vi "Force_1_R2.vi"() -> ()   [LabVIEW 2020]
uses:
  Support/Controls/Cmd_Mouse Popup.ctl
  Support/Controls/Clst_Initialize Input.ctl
  Support/Controls/Clst_Result inspec.ctl
  Support/Controls/Cmd_Var Data IO.ctl
  Variables/Global_Cal Info.vi
panel:
  out "Creep Test_ADJ":string[][](table) caption="2. 영점출력"
  in  "zero_30_ADJ":string[][](table) caption="2. 영점출력"
  in  "zero_300_ADJ":string[][](table) caption="2. 영점출력"
  in  "Measured_ADJ":string[][](table) caption="● 힘 측정기 지시값 (조정후)"
  out "지시단위":string="무차원"
  out "최대지시값":string
  in  "측정방향":string(combo)="인장"
  out "Creep Test":string[][](table) caption="2. 영점출력"
  in  "Case":enum16{"", "Case B", "Case D"}(ring)
  in  "zero_30":string[][](table) caption="2. 영점출력"
  in  "zero_300":string[][](table) caption="2. 영점출력"
  in  "Indicator info":string[][](table) caption="1. 사용 인디케이터"
  out "분해능":string
  out "표시방식":string
  in  "Spec 변경":bool
  in  "Random":bool
  out "Spec":string[][](table)
  out "제목":string
  out "에러 출력":errorcluster
  out "Condition":string[][](table) caption="3. 교정결과"
  in  "최소눈금":string(combo)
  out "단위":string
  out "최대용량":string
  in  "Measured":string[][](table) caption="● 힘 측정기 지시값"
  out "Load?":bool
  # "2. 영점출력 (조정후)"
  # "2. 영점출력"
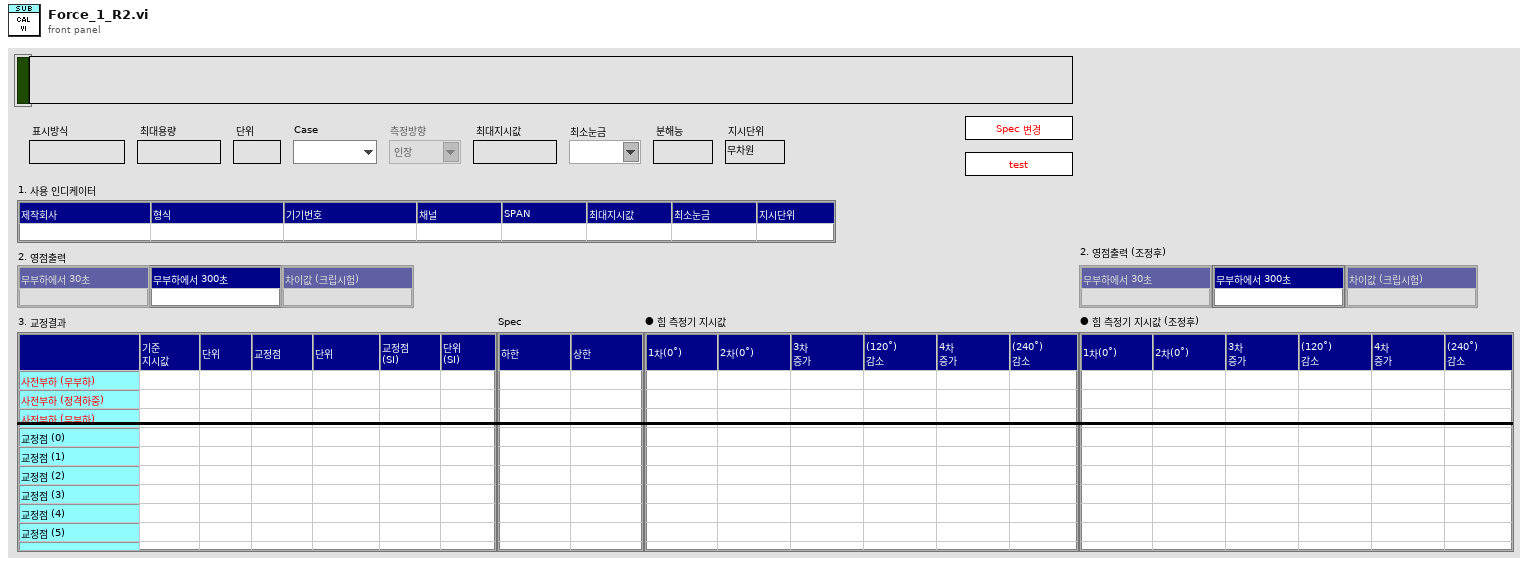
[diagram p1: front panel]
types:
  T1 = typedef "Cmd_Mouse Popup.ctl" = enum16{"활성화", "메뉴선택"}
  T2 = cluster{"Shift":bool, "Ctrl":bool, "Alt":bool, "Cmd":bool, "Opt":bool}
  T3 = enum8{"Enabled", "Disabled", "Disabled and Grayed Out"}
  T4 = typedef "Clst_Initialize Input.ctl" = cluster{"Initialize 1":cluster{"Condition":refnum<vi>[], "Spec":refnum<vi>[], "Measured":refnum<vi>[], "Resolution":refnum<vi>[], "Func_ext":string, "제목":refnum<vi>, "Measured_ADJ":refnum<vi>[]}, "Initialize 2":cluster{"문자열":refnum<vi>[], "콤보박스":refnum<vi>[], "링":refnum<vi>[], "열거형":refnum<vi>[], "테이블":refnum<vi>[], "여러열":refnum<vi>[], "디지털(DBL)":refnum<vi>[], "3D string":refnum<vi>[], "ctrl":refnum<vi>[], "boolean":refnum<vi>[]}}
  T5 = typedef "Clst_Result inspec.ctl" = cluster{"분해능":string, "문자열 1":string, "문자열 2":string, "숫자형 1":i32, "숫자형 2":i32, "숫자형 3":dbl, "문자배열 1D":string[], "문자배열 2D":string[][], "문자배열 3D":string[][][], "문자배열 4D":string[][][][], "불리언 1D":bool[]}
  T6 = typedef "Cmd_Var Data IO.ctl" = enum16{"Condition", "Condition Default", "Condition_Temp", "Resolution", "Resolution Default", "Resolution Old", "Spec", "Spec Default", "Spec Old", "Spec Temp", "Result", "Result2", "Result3", "Result_Temp", "Result_ADJ", "Result_ADJ2", "STD1", "STD2", "STD3", "STD4", "STD5", "STD Temp", "CMC", "CMC Default"}
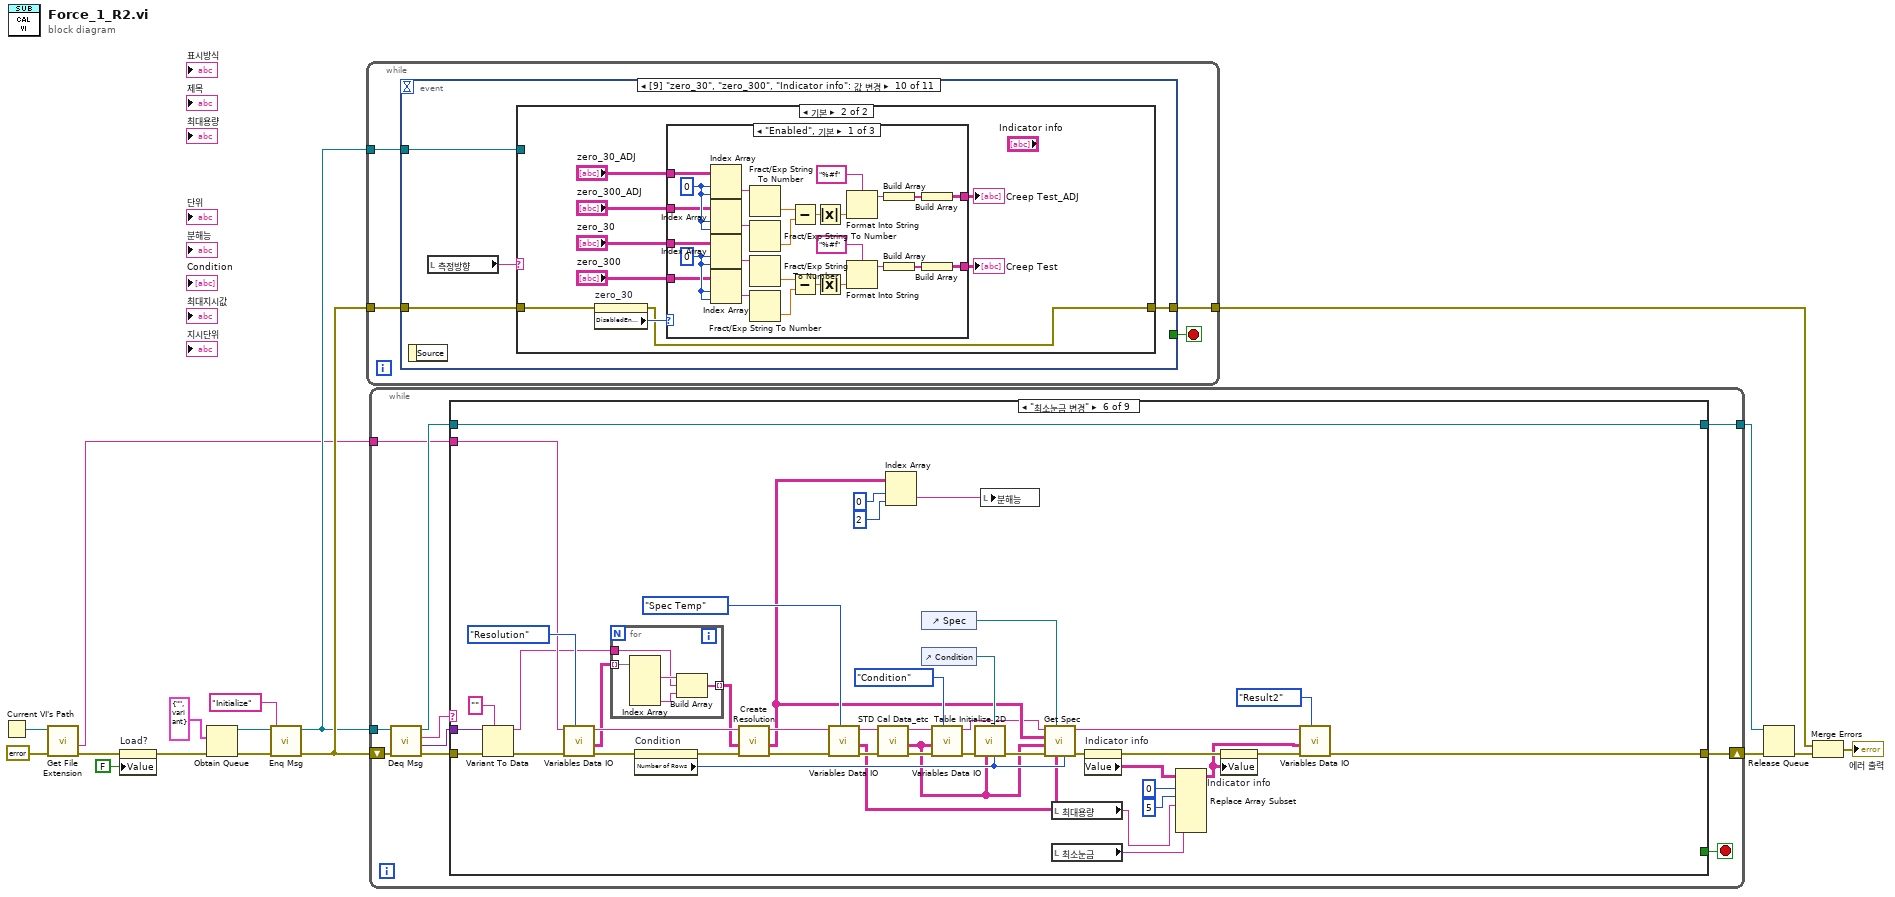
[diagram p0: block diagram]
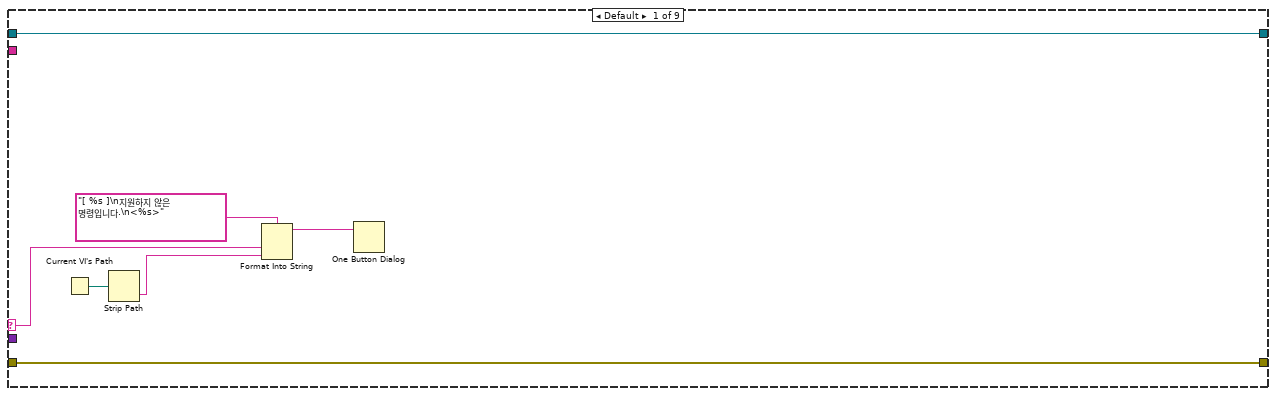
[diagram p2: hidden frame]
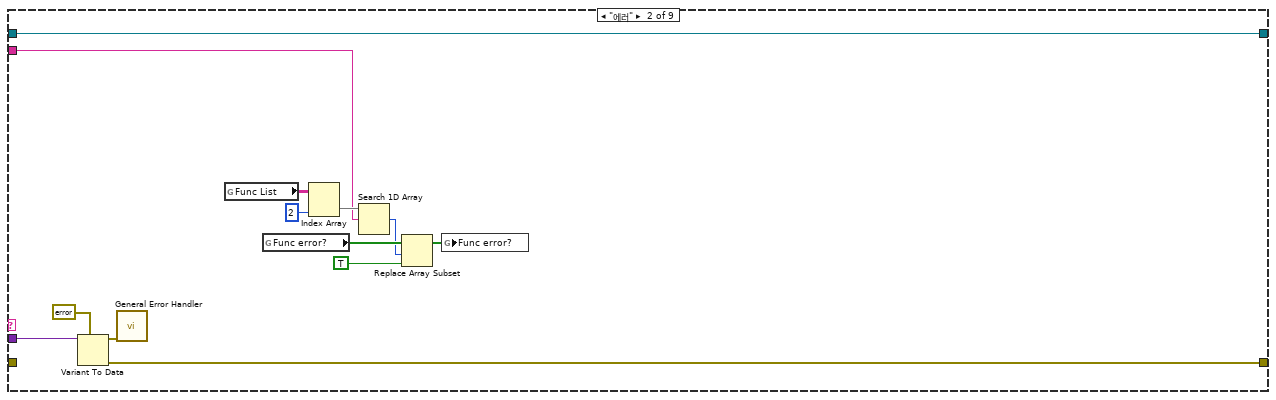
[diagram p3: hidden frame]
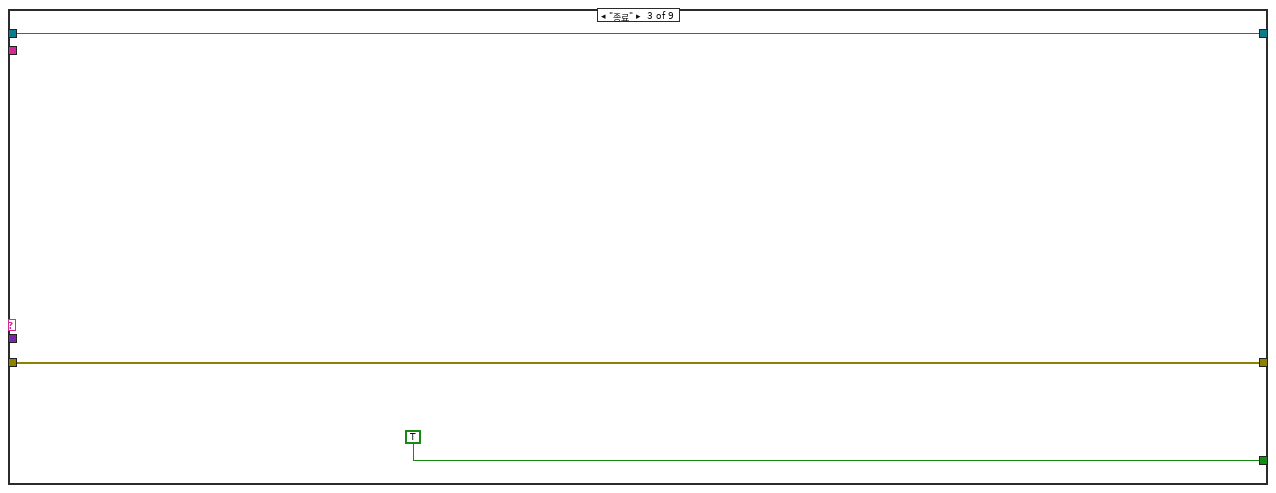
[diagram p4: hidden frame]
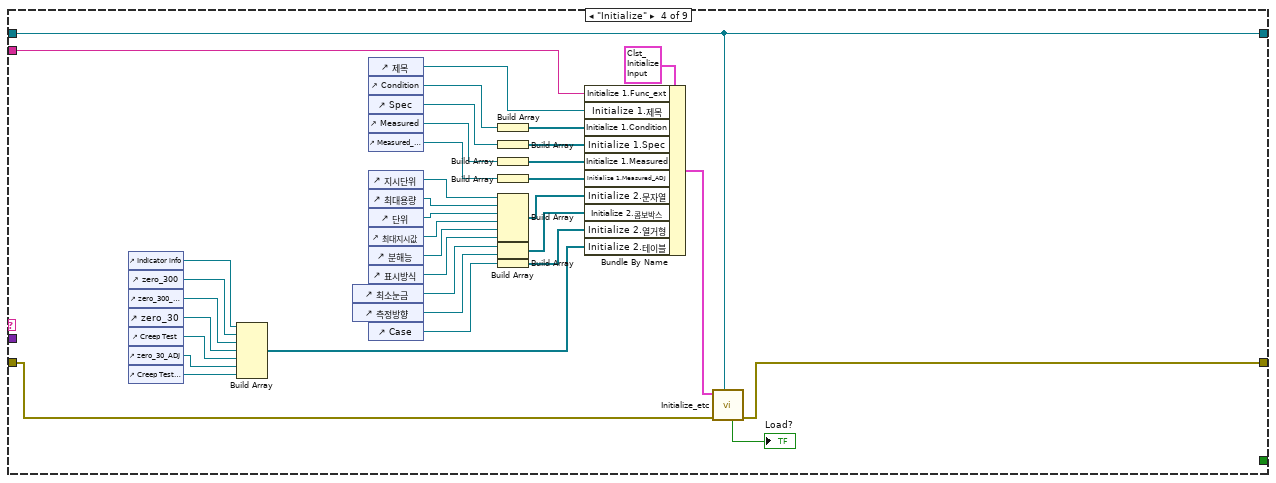
[diagram p5: hidden frame]
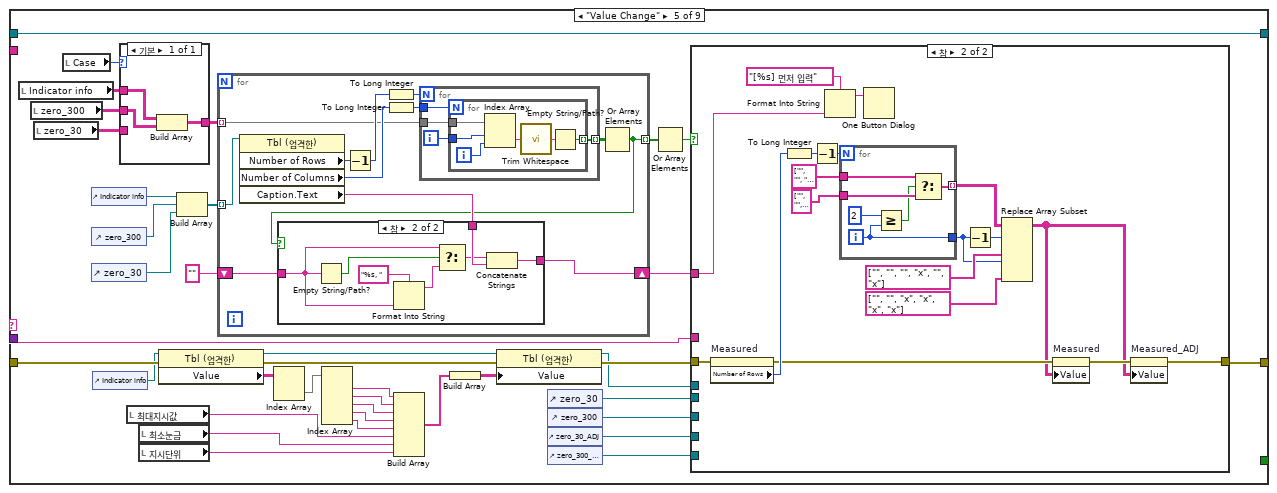
[diagram p6: hidden frame]
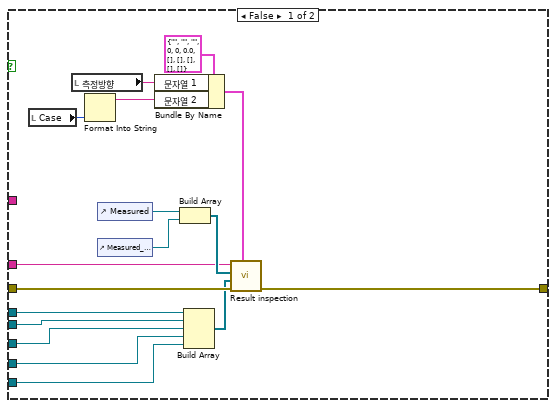
[diagram p7: hidden frame]
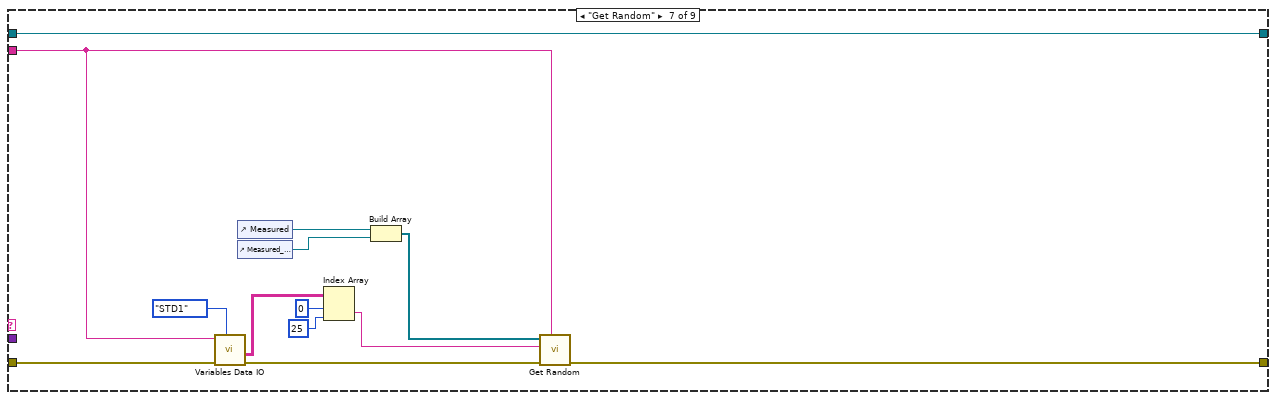
[diagram p9: hidden frame]
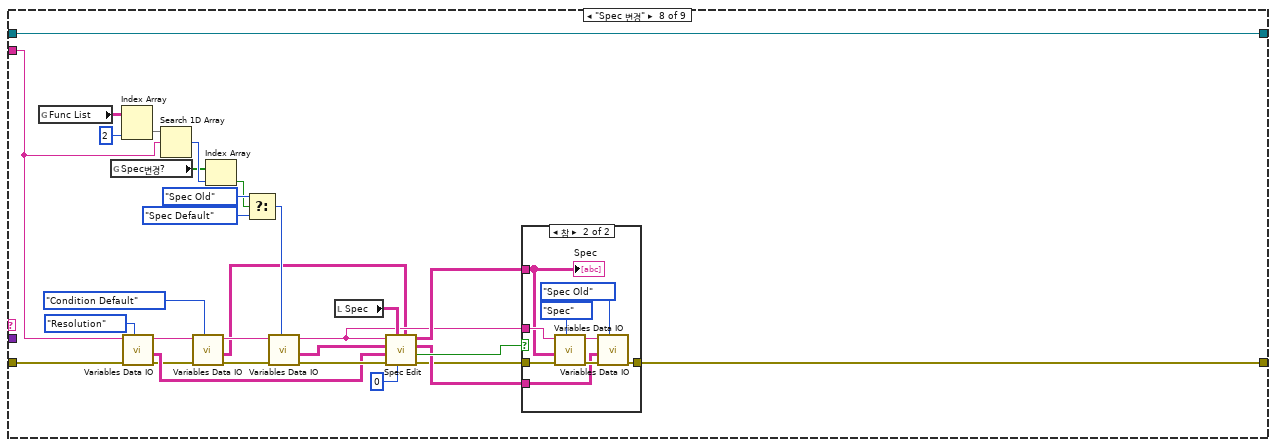
[diagram p10: hidden frame]
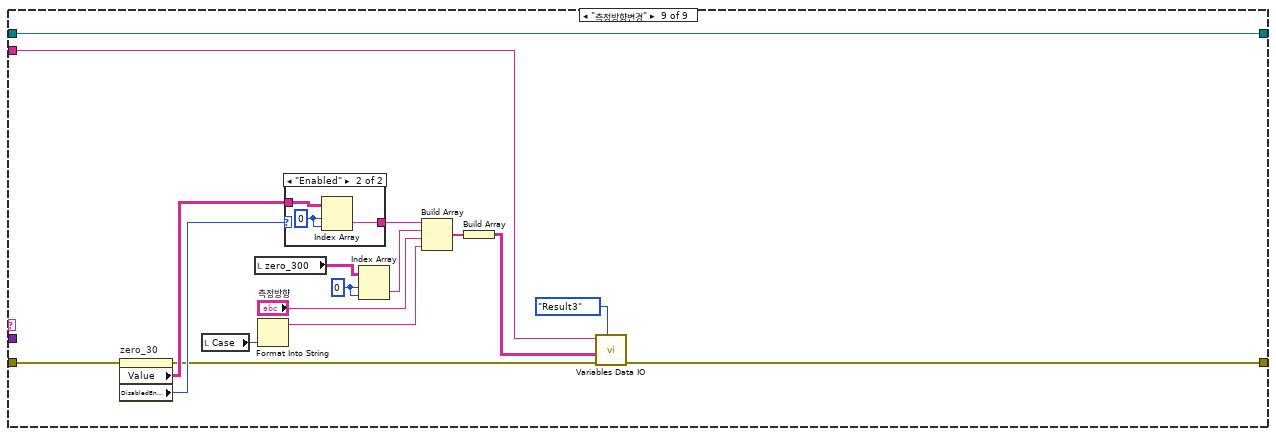
[diagram p12: hidden frame]
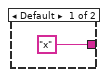
[diagram p13: hidden frame]
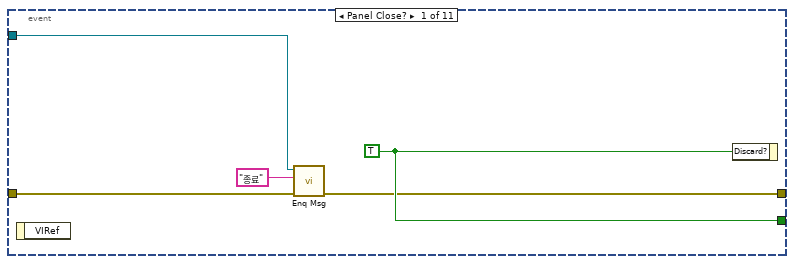
[diagram p14: hidden frame]
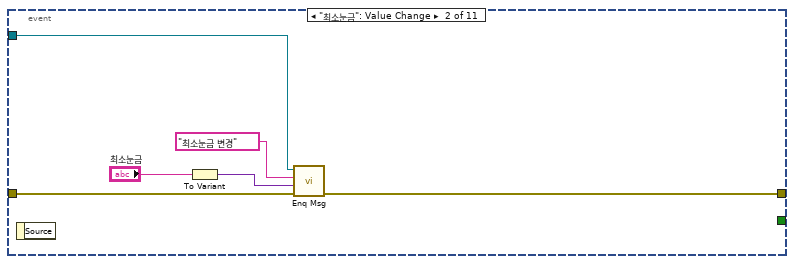
[diagram p15: hidden frame]
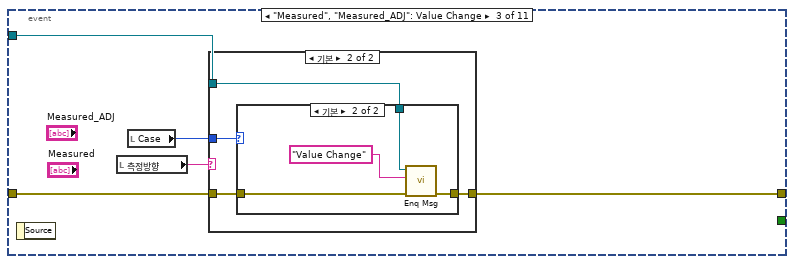
[diagram p16: hidden frame]
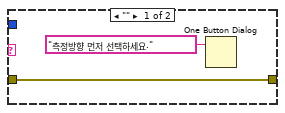
[diagram p17: hidden frame]
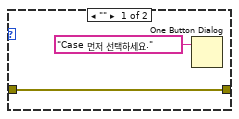
[diagram p18: hidden frame]
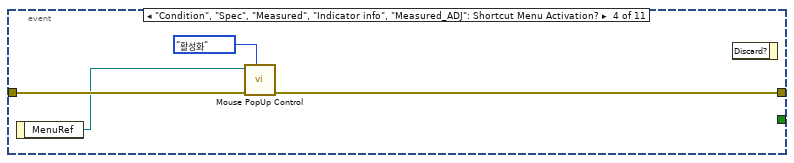
[diagram p19: hidden frame]
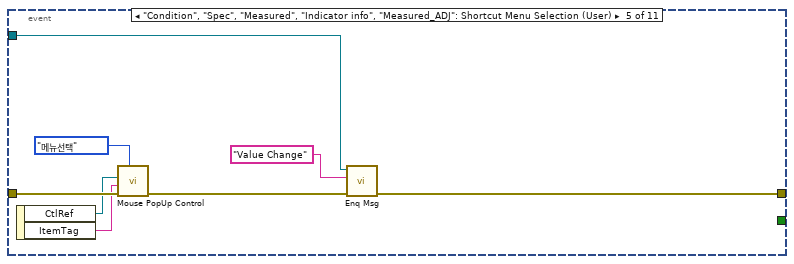
[diagram p20: hidden frame]
diagram:
  n1 = Current VI's Path() -> (path=w5:path)
  n2 = call <vilib>:"Get File Extension.vi"("error in (no error)"=errorcluster {"status"=FALSE, "code"=0, "source"=""} ("에러 상수"), "file"=w5) -> ("error out"=w3:errorcluster, "filename without extension"=w4:string)  [unwired: 5 in, 3 out]
  n3 = property on="Load?" class="Bool (엄격한)"(error in=w3, "Value"=FALSE ("Load?")) -> (error out=w2:errorcluster)  [unwired: 1 in, 1 out]
  n4 = Obtain Queue(element data type=cluster{"메세지":string, "값":variant} {"메세지"="", "값"=variant} ("Message Cluster"), error in (no error)=w2) -> (queue out=w14:refnum<queue>, error out=w16:errorcluster)  [unwired: 3 in, 1 out]
  n5 = call "Enq Msg.vi"("에러 입력(에러 없음)"=w16, "메세지"="Initialize", "큐 입력"=w14) -> ("에러 출력"=w15:errorcluster, "큐 출력"=w12:refnum<queue>)  [unwired: 7 in]
  n6 = while {
    tunnel: w15 -> [w19]
    tunnel: w12 -> [w20]
    tunnel: [w18] -> w9
    stop <- w21 stop-if-true
    n7 = event shown="[9] \"zero_30\", \"zero_300\", \"Indicator info\": 값 변경" {
      selector: _ -> [_ _ _ _ _ _ _ _ _ _ _]
      dyn-events: _ -> [_ _ _ _ _ _ _ _ _ _ _]
      timeout: _ -> [_ _ _ _ _ _ _ _ _ _ _]
      tunnel: [w26 _ _ _ _ _ _ _ _ _ _] -> w21
      tunnel: w20 -> [w24 w31 w36 _ w55 _ w69 w75 w81 w84 w124]
      tunnel: w19 -> [w25 w32 w37 w52 w60 w67 w70 w77 w80 w86 w126]
      tunnel: [w22 w29 w35 w51 w54 w66 w68 w76 w79 w85 w125] -> w18
      event Panel Close? {
        w26 = TRUE ("버림?")
        n8 = event-data() -> ()  [unwired: 1 in, 1 out]
        n9 = call "Enq Msg.vi"("에러 입력(에러 없음)"=w25, "메세지"="종료", "큐 입력"=w24) -> ("에러 출력"=w22:errorcluster)  [unwired: 7 in, 1 out]
        n10 = event-data("Discard?"=w26) -> ()  [unwired: 1 in, 1 out]
      }
      event "최소눈금": Value Change {
        n11 = event-data() -> ()  [unwired: 1 in, 1 out]
        n12 = To Variant(anything="최소눈금") -> (Variant=w27:variant)
        n13 = call "Enq Msg.vi"("에러 입력(에러 없음)"=w32, "값"=w27, "메세지"="최소눈금 변경", "큐 입력"=w31) -> ("에러 출력"=w29:errorcluster)  [unwired: 6 in, 1 out]
      }
      event "Measured", "Measured_ADJ": Value Change {
        n14 = event-data() -> ()  [unwired: 1 in, 1 out]
        n15 = local read "측정방향"() -> (w34:string)
        n16 = local read "Case"() -> (w33:enum16{"", "Case B", "Case D"})
        n17 = case shown="기본" w34 {
          tunnel: w37 -> [w39 w43]
          tunnel: w36 -> [_ w42]
          tunnel: [w39 w41] -> w35
          tunnel: w33 -> [_ w40]
          frame "" {
            n18 = One Button Dialog(message="측정방향 먼저 선택하세요." ("메시지")) -> ()  [unwired: 1 in, 1 out]
          }
          frame Default {
            n19 = case shown="기본" w40 {
              tunnel: w43 -> [w44 w49]
              tunnel: w42 -> [_ w48]
              tunnel: [w44 w46] -> w41
              frame "" {
                n20 = One Button Dialog(message="Case 먼저 선택하세요." ("메시지")) -> ()  [unwired: 1 in, 1 out]
              }
              frame Default {
                n21 = call "Enq Msg.vi"("에러 입력(에러 없음)"=w49, "메세지"="Value Change", "큐 입력"=w48) -> ("에러 출력"=w46:errorcluster)  [unwired: 7 in, 1 out]
              }
            }
          }
        }
      }
      event "Condition", "Spec", "Measured", "Indicator info", "Measured_ADJ": Shortcut Menu Activation? {
        n22 = event-data() -> ("MenuRef"=w50:refnum<k9>)  [unwired: 1 in]
        n23 = call "Mouse PopUp Control.vi"("type"=Cmd_Mouse_Popup."활성화", "error in"=w52, "메뉴 참조"=w50) -> ("error out"=w51:errorcluster)  [unwired: 8 in]
        n24 = event-data() -> ()  [unwired: 2 in, 1 out]
      }
      event "Condition", "Spec", "Measured", "Indicator info", "Measured_ADJ": Shortcut Menu Selection (User) {
        n25 = event-data() -> ("CtlRef"=w58:refnum<vi>, "ItemTag"=w59:string)  [unwired: 1 in]
        n26 = call "Mouse PopUp Control.vi"("type"=Cmd_Mouse_Popup."메뉴선택", "error in"=w60, "아이템 태그"=w59, "Tbl 참조 번호"=w58) -> ("error out"=w56:errorcluster)  [unwired: 7 in]
        n27 = call "Enq Msg.vi"("에러 입력(에러 없음)"=w56, "메세지"="Value Change", "큐 입력"=w55) -> ("에러 출력"=w54:errorcluster)  [unwired: 7 in, 1 out]
      }
      event "Measured", "Indicator info", "Condition", "Measured_ADJ": Key Down; "Measured", "Indicator info", "Condition", "Measured_ADJ": Key Repeat {
        n28 = event-data() -> ("PlatMods"=w62:T2, "ScanCode"=w65:i16, "Mods.Num Pad"=w64:bool, "CtlRef"=w63:refnum<vi>)  [unwired: 1 in]
        n29 = call "Cursor Control.vi"("플랫폼 조합키"=w62, "참조"=w63, "Num Pad"=w64, "ScanCode"=w65, "error in"=w67) -> ("error out"=w66:errorcluster)  [unwired: 5 in, 1 out]
      }
      event "Random": Value Change {
        n30 = event-data() -> ()  [unwired: 1 in, 1 out]
        n31 = call "Enq Msg.vi"("에러 입력(에러 없음)"=w70, "메세지"="Get Random", "큐 입력"=w69) -> ("에러 출력"=w72:errorcluster, "큐 출력"=w73:refnum<queue>)  [unwired: 7 in]
        n32 = call "Enq Msg.vi"("에러 입력(에러 없음)"=w72, "메세지"="Value Change", "큐 입력"=w73) -> ("에러 출력"=w68:errorcluster)  [unwired: 7 in, 1 out]
      }
      event "Spec 변경": Value Change {
        n33 = event-data() -> ()  [unwired: 1 in, 1 out]
        n34 = call "Enq Msg.vi"("에러 입력(에러 없음)"=w77, "메세지"="Spec 변경", "큐 입력"=w75) -> ("에러 출력"=w76:errorcluster)  [unwired: 7 in, 1 out]
      }
      event "Case": Value Change {
        n35 = event-data() -> ()  [unwired: 1 in, 1 out]
        n36 = call "Enq Msg.vi"("에러 입력(에러 없음)"=w80, "메세지"="Value Change", "큐 입력"=w81) -> ("에러 출력"=w79:errorcluster)  [unwired: 7 in, 1 out]
      }
      event "zero_30", "zero_300", "Indicator info": Value Change {
        n37 = event-data() -> ()  [unwired: 1 in, 1 out]
        n38 = local read "측정방향"() -> (w83:string)
        n39 = case shown="기본" w83 {
          tunnel: w86 -> [w88 w95]
          tunnel: [w88 w92] -> w85
          tunnel: w84 -> [_ _]
          frame "" {
            n40 = One Button Dialog(message="측정방향 먼저 선택하세요." ("메시지")) -> ()  [unwired: 1 in, 1 out]
          }
          frame Default {
            n41 = property on="zero_30" class="Tbl (엄격한)"(error in=w95) -> (error out=w92:errorcluster, "DisabledEnum"=w94:T3)  [unwired: 1 in, 1 out]
            n42 = case shown="\"Enabled\", 기본" w94 {
              tunnel: "zero_30" -> [w122 _ _]
              tunnel: "zero_300" -> [w120 _ _]
              tunnel: [w112 _ _] -> w93
              tunnel: "zero_30_ADJ" -> [w100 _ _]
              tunnel: "zero_300_ADJ" -> [w99 _ _]
              tunnel: [w98 _ _] -> w89
              frame "Enabled", Default {
                w101 = 0 ("인덱스 (행)")
                w123 = 0 ("인덱스 (행)")
                n43 = Index Array(array=w100, index (row)=w101, index (col)=w101) -> (element=w105:string)
                n44 = Index Array(array=w99, index (row)=w101, index (col)=w101) -> (element=w106:string)
                n45 = Index Array(array=w122, index (row)=w123, index (col)=w123) -> (element=w117:string)
                n46 = Index Array(array=w120, index (row)=w123, index (col)=w123) -> (element=w116:string)
                n47 = Fract/Exp String To Number(string=w105) -> (number=w102:dbl)  [unwired: 3 in, 1 out]
                n48 = Fract/Exp String To Number(string=w106) -> (number=w103:dbl)  [unwired: 3 in, 1 out]
                n49 = Fract/Exp String To Number(string=w117) -> (number=w121:dbl)  [unwired: 3 in, 1 out]
                n50 = Fract/Exp String To Number(string=w116) -> (number=w119:dbl)  [unwired: 3 in, 1 out]
                n51 = Subtract(x=w102, y=w103) -> (x-y=w104:dbl)
                n52 = Subtract(x=w121, y=w119) -> (x-y=w118:dbl)
                n53 = Absolute Value(x=w104) -> (abs(x)=w110:dbl)
                n54 = Absolute Value(x=w118) -> (abs(x)=w111:dbl)
                n55 = Format Into String(format string="%#f" ("포맷 문자열"), w110) -> (resulting string=w108:string)  [unwired: 2 in, 1 out]
                n56 = Format Into String(format string="%#f" ("포맷 문자열"), w111) -> (resulting string=w114:string)  [unwired: 2 in, 1 out]
                n57 = Build Array(w108) -> (w109:string[])
                n58 = Build Array(w114) -> (w113:string[])
                n59 = Build Array(w109) -> (w98:string[][])
                n60 = Build Array(w113) -> (w112:string[][])
              }
              frame "Disabled" {
              }
              frame "Disabled and Grayed Out" {
              }
            }
            "Creep Test" <- w93
            "Creep Test_ADJ" <- w89
          }
        }
      }
      event "측정방향": Value Change {
        n61 = event-data() -> ()  [unwired: 1 in, 1 out]
        n62 = call "Enq Msg.vi"("에러 입력(에러 없음)"=w126, "메세지"="측정방향변경", "큐 입력"=w124) -> ("에러 출력"=w125:errorcluster)  [unwired: 7 in, 1 out]
      }
    }
  }
  n63 = while {
    shift-right: [w137] -> w11
    shift-left: w15 -> [w136]
    tunnel: w12 -> [w134]
    tunnel: [w129] -> w10
    tunnel: w4 -> [w128]
    stop <- w130 stop-if-true
    n64 = call "Deq Msg.vi"("에러 입력(에러 없음)"=w136, "큐 입력"=w134) -> ("에러 출력"=w135:errorcluster, "값"=w131:variant, "메세지"=w133:string, "큐 출력"=w132:refnum<queue>)  [unwired: 6 in]
    n65 = case shown="\"최소눈금 변경\"" w133 {
      selector: w133 -> [w140 _ _ _ _ _ _ _ _]
      tunnel: w135 -> [w144 _ w160 w175 w216 w352 w366 w381 w414]
      tunnel: [w144 w154 w160 w180 w225 w316 w369 w382 w426] -> w137
      tunnel: w132 -> [w143 w153 w158 w184 w234 w353 w371 w401 w428]
      tunnel: w131 -> [_ w155 _ _ _ w351 _ _ _]
      tunnel: [_ _ TRUE ("버림?") _ _ _ _ _ _] -> w130
      tunnel: [w143 w153 w158 w184 w234 w353 w371 w401 w428] -> w129
      tunnel: w128 -> [_ w145 _ w179 w224 w347 w367 w380 w425]
      frame Default {
        n66 = Current VI's Path() -> (path=w139:path)
        n67 = Strip Path(path=w139) -> (name=w138:string)  [unwired: 1 out]
        n68 = Format Into String(format string="[ %s ]\n지원하지 않은 명령입니다.\n<%s>" ("메시지"), w140, w138) -> (resulting string=w141:string)  [unwired: 2 in, 1 out]
        n69 = One Button Dialog(message=w141) -> ()  [unwired: 1 in, 1 out]
      }
      frame "에러" {
        n70 = Variant To Data(type=errorcluster {"status"=FALSE, "code"=0, "source"=""} ("에러 출력"), Variant=w155) -> (data=w157:errorcluster, error out=w154:errorcluster)  [unwired: 1 in]
        n71 = call <vilib>:"General Error Handler.vi"("error in (no error)"=w157) -> ()  [unwired: 10 in, 5 out]
        n72 = global read "Global_Cal Info.vi" "Func List"() -> (w151:string[][])
        n73 = global read "Global_Cal Info.vi" "Func error?"() -> (w148:bool[])
        n74 = Index Array(array=w151, index (col)=2 ("비활성화된 인덱스 (열)")) -> (element=w150:string[])  [unwired: 1 in]
        n75 = Search 1D Array(1D array=w150, element=w145) -> (index of element=w147:i32)  [unwired: 1 in]
        n76 = Replace Array Subset(array=w148, new element=TRUE ("새 원소/부분배열"), index=w147) -> (w146:bool[])
        n77 = global write "Global_Cal Info.vi" "Func error?"(w146) -> ()
      }
      frame "종료" {
      }
      frame "Initialize" {
        n78 = control-ref of="Indicator info"() -> (w174:refnum<vi>)
        n79 = control-ref of="zero_300"() -> (w173:refnum<vi>)
        n80 = control-ref of="zero_300_ADJ"() -> (w165:refnum<vi>)
        n81 = control-ref of="zero_30"() -> (w164:refnum<vi>)
        n82 = control-ref of="Creep Test"() -> (w163:refnum<vi>)
        n83 = control-ref of="zero_30_ADJ"() -> (w162:refnum<vi>)
        n84 = control-ref of="Creep Test_ADJ"() -> (w166:refnum<vi>)
        n85 = Build Array(w174, w173, w165, w164, w163, w162, w166) -> (w172:refnum<vi>[])
        n86 = control-ref of="최소눈금"() -> (w190:refnum<vi>)
        n87 = control-ref of="측정방향"() -> (w171:refnum<vi>)
        n88 = control-ref of="제목"() -> (w188:refnum<vi>)
        n89 = control-ref of="Condition"() -> (w183:refnum<vi>)
        n90 = control-ref of="Spec"() -> (w182:refnum<vi>)
        n91 = control-ref of="Measured"() -> (w192:refnum<vi>)
        n92 = control-ref of="Measured_ADJ"() -> (w167:refnum<vi>)
        n93 = control-ref of="지시단위"() -> (w169:refnum<vi>)
        n94 = control-ref of="최대용량"() -> (w187:refnum<vi>)
        n95 = control-ref of="단위"() -> (w178:refnum<vi>)
        n96 = control-ref of="최대지시값"() -> (w186:refnum<vi>)
        n97 = control-ref of="분해능"() -> (w181:refnum<vi>)
        n98 = control-ref of="표시방식"() -> (w170:refnum<vi>)
        n99 = control-ref of="Case"() -> (w177:refnum<vi>)
        n100 = Build Array(w183) -> (w194:refnum<vi>[])
        n101 = Build Array(w182) -> (w185:refnum<vi>[])
        n102 = Build Array(w192) -> (w193:refnum<vi>[])
        n103 = Build Array(w167) -> (w168:refnum<vi>[])
        n104 = Build Array(w169, w187, w178, w186, w181, w170) -> (w191:refnum<vi>[])
        n105 = Build Array(w190, w171) -> (w189:refnum<vi>[])
        n106 = Build Array(w177) -> (w176:refnum<vi>[])
        n107 = Bundle By Name(cluster=T4 {"Initialize 1"={"Condition"=[], "Spec"=[], "Measured"=[], "Resolution"=[], "Func_ext"="", "제목"=refnum, "Measured_ADJ"=[]}, "Initialize 2"={"문자열"=[], "콤보박스"=[], "링"=[], "열거형"=[], "테이블"=[], "여러열"=[], "디지털(DBL)"=[], "3D string"=[], "ctrl"=[], "boolean"=[]}} ("입력 클러스터"), "Initialize 1.Func_ext"=w179, "Initialize 1.제목"=w188, "Initialize 1.Condition"=w194, "Initialize 1.Spec"=w185, "Initialize 1.Measured"=w193, "Initialize 1.Measured_ADJ"=w168, "Initialize 2.문자열"=w191, "Initialize 2.콤보박스"=w189, "Initialize 2.열거형"=w176, "Initialize 2.테이블"=w172) -> (w195:T4)
        n108 = call "Initialize_etc.vi"("큐 입력"=w184, "error in"=w175, "입력 클러스터"=w195) -> ("error out"=w180:errorcluster, "Load?"=→"Load?":bool)  [unwired: 6 in, 1 out]
      }
      frame "Value Change" {
        n109 = local read "Indicator info"() -> (w217:string[][])
        n110 = local read "zero_300"() -> (w220:string[][])
        n111 = local read "zero_30"() -> (w221:string[][])
        n112 = local read "Case"() -> (w232:enum16{"", "Case B", "Case D"})
        n113 = control-ref of="Indicator info"() -> (w230:refnum<vi>)
        n114 = control-ref of="zero_300"() -> (w229:refnum<vi>)
        n115 = control-ref of="zero_30"() -> (w228:refnum<vi>)
        n116 = control-ref of="Indicator info"() -> (w212:refnum<vi>)
        n117 = case shown="기본" w232 {
          tunnel: w217 -> [w278]
          tunnel: w220 -> [w277]
          tunnel: w221 -> [_]
          tunnel: [w276] -> w231
          frame 기본 {
            n118 = Build Array(w278, w277) -> (w276:string[][][])
          }
        }
        n119 = local read "최대지시값"() -> (w203:string)
        n120 = local read "최소눈금"() -> (w202:string)
        n121 = local read "지시단위"() -> (w201:string)
        n122 = property on="프로퍼티 노드" class="Tbl (엄격한)"(reference=w212, error in=w216) -> (reference out=w213:refnum<vi>, error out=w215:errorcluster, "Value"=w210:string[][])
        n123 = Build Array(w230, w229, w228) -> (w227:refnum<vi>[])
        n124 = for {
          tunnel: w227 -> [w290] mode=indexing
          tunnel: w231 -> [w286] mode=indexing
          tunnel: [w279] -> w233 mode=indexing
          shift-right: [w283] -> w222
          shift-left: "" -> [w284]
          n125 = property on="프로퍼티 노드" class="Tbl (엄격한)"(reference=w290) -> ("Number of Rows"=w289:u32, "Number of Columns"=w288:u32, "Caption.Text"=w285:string)  [unwired: 1 in, 2 out]
          n126 = Decrement(x=w289) -> (x-1=w287:u32)
          n127 = To Long Integer(number=w287) -> (32bit integer=w282:i32)
          n128 = To Long Integer(number=w288) -> (32bit integer=w281:i32)
          n129 = for {
            N: w282 -> [_]
            tunnel: w286 -> [w301]
            tunnel: w281 -> [w302]
            tunnel: [w300] -> w280 mode=indexing
            i -> [w299]
            n130 = for {
              N: w302 -> [_]
              tunnel: w301 -> [w306]
              tunnel: [w307] -> w300 mode=indexing
              tunnel: w299 -> [w304]
              i -> [w303]
              n131 = Index Array(array=w306, index (row)=w304, index (col)=w303) -> (element=w305:string)
              n132 = call <vilib>:"Trim Whitespace.vi"("string"=w305) -> ("trimmed string"=w308:string)  [unwired: 1 in]
              n133 = Empty String/Path?(string/path=w308) -> (empty?=w307:bool)
            }
          }
          n134 = Or Array Elements(Boolean array=w280) -> (logical OR=w279:bool)
          n135 = case shown="참" w279 {
            tunnel: w285 -> [_ w298]
            tunnel: w284 -> [w291 w297]
            tunnel: [w291 w296] -> w283
            frame False {
            }
            frame True {
              n136 = Empty String/Path?(string/path=w297) -> (empty?=w295:bool)
              n137 = Format Into String(format string="%s, " ("포맷 문자열"), w297) -> (resulting string=w293:string)  [unwired: 2 in, 1 out]
              n138 = Select(t=w297, s=w295, f=w293) -> (s? t:f=w292:string)
              n139 = Concatenate Strings(w292, w298) -> (w296:string)
            }
          }
        }
        n140 = Index Array(array=w210) -> (element=w209:string[])  [unwired: 2 in]
        n141 = Index Array(array=w209) -> (element #1=w208:string, element #2=w207:string, element #3=w206:string, element #4=w205:string, element #5=w204:string)  [unwired: 5 in]
        n142 = Build Array(w208, w207, w206, w205, w204, w203, w202, w201) -> (w200:string[])
        n143 = Build Array(w200) -> (w199:string[][])
        n144 = property on="프로퍼티 노드" class="Tbl (엄격한)"(reference=w213, error in=w215, "Value"=w199) -> (reference out=w211:refnum<vi>, error out=w214:errorcluster)
        n145 = control-ref of="zero_30"() -> (w219:refnum<vi>)
        n146 = control-ref of="zero_300"() -> (w218:refnum<vi>)
        n147 = control-ref of="zero_30_ADJ"() -> (w198:refnum<vi>)
        n148 = control-ref of="zero_300_ADJ"() -> (w197:refnum<vi>)
        n149 = Or Array Elements(Boolean array=w233) -> (logical OR=w223:bool)
        n150 = case shown="참" w223 {
          tunnel: [w251 w253] -> w225
          tunnel: w214 -> [w250 w266]
          tunnel: w224 -> [w247 _]
          tunnel: w222 -> [_ w267]
          tunnel: w211 -> [w246 _]
          tunnel: w219 -> [w245 _]
          tunnel: w218 -> [w244 _]
          tunnel: w198 -> [w236 _]
          tunnel: w197 -> [w235 _]
          frame False {
            n151 = local read "Case"() -> (w239:enum16{"", "Case B", "Case D"})
            n152 = local read "측정방향"() -> (w240:string)
            n153 = Format Into String(w239) -> (resulting string=w238:string)  [unwired: 3 in, 1 out]
            n154 = control-ref of="Measured"() -> (w249:refnum<vi>)
            n155 = control-ref of="Measured_ADJ"() -> (w237:refnum<vi>)
            n156 = Bundle By Name(cluster=T5 {"분해능"="", "문자열 1"="", "문자열 2"="", "숫자형 1"=0, "숫자형 2"=0, "숫자형 3"=0.0, "문자배열 1D"=[], "문자배열 2D"=[], "문자배열 3D"=[], "문자배열 4D"=[], "불리언 1D"=[]} ("입력 클러스터"), "문자열 1"=w240, "문자열 2"=w238) -> (w241:T5)
            n157 = Build Array(w249, w237) -> (w248:refnum<vi>[])
            n158 = Build Array(w246, w245, w244, w236, w235) -> (w243:refnum<vi>[])
            n159 = call "Result inspection.vi"("입력 클러스터"=w241, "error in"=w250, "Ref. Data (excluded)"=w243, "Ref. Data (Inspection)"=w248, "Func ext"=w247) -> ("error out"=w251:errorcluster)  [unwired: 3 in, 3 out]
          }
          frame True {
            n160 = property on="Measured" class="Tbl (엄격한)"(error in=w266) -> (error out=w255:errorcluster, "Number of Rows"=w256:u32)  [unwired: 1 in, 1 out]
            n161 = To Long Integer(number=w256) -> (32bit integer=w264:i32)
            n162 = Decrement(x=w264) -> (x-1=w265:i32)
            n163 = Format Into String(format string="[%s] 먼저 입력" ("포맷 문자열"), w267) -> (resulting string=w269:string)  [unwired: 2 in, 1 out]
            n164 = for {
              N: w265 -> [_]
              tunnel: [w272] -> w257 mode=indexing
              tunnel: [w275] -> w259
              tunnel: string[] ["", "", "", "", "", ""] -> [w274]
              tunnel: string[] ["", "", "", "ⅹ", "ⅹ", "ⅹ"] -> [w273]
              i -> [w275]
              n165 = Greater Or Equal?(x=2, y=w275) -> (x >= y?=w271:bool)
              n166 = Select(t=w273, s=w271, f=w274) -> (s? t:f=w272:string[])
            }
            n167 = One Button Dialog(message=w269) -> ()  [unwired: 1 in, 1 out]
            n168 = Decrement(x=w259) -> (x-1=w260:i32)
            n169 = Replace Array Subset(array=w257, new element #1=string[] ["", "", "", "ⅹ", "", "ⅹ"], index (row) #1=w260, new element #2=string[] ["", "", "ⅹ", "ⅹ", "ⅹ", "ⅹ"], index (row) #2=w259) -> (w252:string[][])  [unwired: 2 in]
            n170 = property on="Measured" class="Tbl (엄격한)"(error in=w255, "Value"=w252) -> (error out=w254:errorcluster)  [unwired: 1 in, 1 out]
            n171 = property on="Measured_ADJ" class="Tbl (엄격한)"(error in=w254, "Value"=w252) -> (error out=w253:errorcluster)  [unwired: 1 in, 1 out]
          }
        }
      }
      frame "최소눈금 변경" {
        n172 = Variant To Data(error in=w352, type="", Variant=w351) -> (data=w345:string, error out=w346:errorcluster)
        n173 = call "Variables Data IO.vi"("Select"=Cmd_Var_Data_IO."Resolution", "error in"=w346, "Func_ext"=w347) -> ("error out"=w331:errorcluster, "Data Out"=w344:string[][], "Func_ext Out"=w348:string)  [unwired: 6 in]
        n174 = for {
          tunnel: w344 -> [w358] mode=indexing
          tunnel: w345 -> [w356]
          tunnel: [w354] -> w343 mode=indexing
          n175 = Index Array(array=w358) -> (element #1=w357:string, element #4=w355:string)  [unwired: 4 in, 2 out]
          n176 = Build Array(w357, w356, w355) -> (w354:string[])
        }
        n177 = property on="Condition" class="Tbl (엄격한)"(error in=w331) -> (error out=w330:errorcluster, "Number of Rows"=w313:u32)  [unwired: 1 in, 1 out]
        n178 = call "Create Resolution.vi"("에러 입력(에러 없음)"=w330, "Resolution"=w343, "Func_ext"=w348) -> ("에러 출력"=w335:errorcluster, "Resolution Out"=w310:string[][], "Func_ext 출력"=w334:string)  [unwired: 6 in]
        n179 = call "Variables Data IO.vi"("Select"=Cmd_Var_Data_IO."Spec Temp", "error in"=w335, "Func_ext"=w334) -> ("error out"=w333:errorcluster, "Data Out"=w312:string[][], "Func_ext Out"=w332:string)  [unwired: 6 in]
        n180 = call "STD Cal Data_etc.vi"("error in"=w333, "Func_ext"=w332) -> ("error out"=w340:errorcluster, "Data Out"=w311:string[][], "Func_ext Out"=w341:string)  [unwired: 5 in, 2 out]
        n181 = Index Array(array=w310, index (row)=0 ("인덱스 (행)"), index (col)=2 ("비활성화된 인덱스 (열)")) -> (element=w327:string)
        n182 = control-ref of="Spec"() -> (w337:refnum<vi>)
        n183 = control-ref of="Condition"() -> (w326:refnum<vi>)
        n184 = call "Variables Data IO.vi"("Select"=Cmd_Var_Data_IO."Condition", "error in"=w340, "Data In"=w311, "Func_ext"=w341) -> ("error out"=w339:errorcluster, "Func_ext Out"=w309:string)  [unwired: 5 in, 1 out]
        n185 = call "Table Initialize_2D.vi"("행의 개수"=w313, "Table Ref"=w326, "Value"=w311, "에러 입력"=w339) -> ("에러 출력"=w342:errorcluster)  [unwired: 5 in, 2 out]
        n186 = local write "분해능"(w327) -> ()
        n187 = call "Get Spec.vi"("NumRows"=w313, "Spec in"=w312, "Spec Ref."=w337, "error in"=w342, "Condition in"=w311, "Resolution in"=w310, "Func_ext"=w309) -> ("error out"=w319:errorcluster, "Func_ext Out"=w315:string)  [unwired: 3 out]
        n188 = local read "최대용량"() -> (w322:string)
        n189 = local read "최소눈금"() -> (w320:string)
        n190 = property on="Indicator info" class="Tbl (엄격한)"(error in=w319) -> (error out=w325:errorcluster, "Value"=w324:string[][])  [unwired: 1 in, 1 out]
        n191 = Replace Array Subset(array=w324, new element #1=w322, index (row) #1=0 ("비활성화된 인덱스 (행)"), index (col) #1=5 ("비활성화된 인덱스 (열)"), new element #2=w320) -> (w314:string[][])  [unwired: 2 in]
        n192 = property on="Indicator info" class="Tbl (엄격한)"(error in=w325, "Value"=w314) -> (error out=w317:errorcluster)  [unwired: 1 in, 1 out]
        n193 = call "Variables Data IO.vi"("Select"=Cmd_Var_Data_IO."Result2", "error in"=w317, "Data In"=w314, "Func_ext"=w315) -> ("error out"=w316:errorcluster)  [unwired: 5 in, 2 out]
      }
      frame "Get Random" {
        n194 = call "Variables Data IO.vi"("Select"=Cmd_Var_Data_IO."STD1", "error in"=w366, "Func_ext"=w367) -> ("error out"=w365:errorcluster, "Data Out"=w363:string[][])  [unwired: 6 in, 1 out]
        n195 = control-ref of="Measured"() -> (w368:refnum<vi>)
        n196 = control-ref of="Measured_ADJ"() -> (w359:refnum<vi>)
        n197 = Index Array(array=w363, index (row)=0 ("인덱스 (행)"), index (col)=25 ("비활성화된 인덱스 (열)")) -> (element=w360:string)
        n198 = Build Array(w368, w359) -> (w370:refnum<vi>[])
        n199 = call "Get Random.vi"("Func_Ext"=w367, "에러 입력"=w365, "분해능"=w360, "Meas"=w370) -> ("에러 출력"=w369:errorcluster)  [unwired: 6 in, 1 out]
      }
      frame "Spec 변경" {
        n200 = global read "Global_Cal Info.vi" "Func List"() -> (w388:string[][])
        n201 = global read "Global_Cal Info.vi" "Spec변경?"() -> (w384:bool[])
        n202 = Index Array(array=w388, index (col)=2 ("비활성화된 인덱스 (열)")) -> (element=w386:string[])  [unwired: 1 in]
        n203 = call "Variables Data IO.vi"("Select"=Cmd_Var_Data_IO."Resolution", "error in"=w381, "Func_ext"=w380) -> ("error out"=w377:errorcluster, "Data Out"=w378:string[][], "Func_ext Out"=w376:string)  [unwired: 6 in]
        n204 = Search 1D Array(1D array=w386, element=w380) -> (index of element=w385:i32)  [unwired: 1 in]
        n205 = call "Variables Data IO.vi"("Select"=Cmd_Var_Data_IO."Condition Default", "error in"=w377, "Func_ext"=w376) -> ("error out"=w374:errorcluster, "Data Out"=w372:string[][], "Func_ext Out"=w375:string)  [unwired: 6 in]
        n206 = Index Array(array=w384, index=w385) -> (element=w389:bool)
        n207 = Select(t=Cmd_Var_Data_IO."Spec Old" ("Select"), s=w389, f=Cmd_Var_Data_IO."Spec Default" ("Select")) -> (s? t:f=w383:T6)
        n208 = call "Variables Data IO.vi"("Select"=w383, "error in"=w374, "Func_ext"=w375) -> ("error out"=w393:errorcluster, "Data Out"=w379:string[][], "Func_ext Out"=w394:string)  [unwired: 6 in]
        n209 = local read "Spec"() -> (w396:string[][])
        n210 = call "Spec Edit.vi"("Condition"=w372, "열번호(기준값)"=0 ("기준열(0)"), "Spec Value"=w396, "에러 입력(에러 없음)"=w393, "Resolution"=w378, "Spec Default"=w379, "Func_ext"=w394) -> ("에러 출력"=w395:errorcluster, "변경?"=w400:bool, "Spec Default out"=w399:string[][], "Spec 출력"=w397:string[][])  [unwired: 1 in]
        n211 = case shown="참" w400 {
          tunnel: w395 -> [w402 w410]
          tunnel: [w402 w407] -> w382
          tunnel: w397 -> [_ w403]
          tunnel: w394 -> [_ w409]
          tunnel: w399 -> [_ w404]
          frame False {
          }
          frame True {
            n212 = call "Variables Data IO.vi"("Select"=Cmd_Var_Data_IO."Spec", "error in"=w410, "Data In"=w403, "Func_ext"=w409) -> ("error out"=w408:errorcluster, "Func_ext Out"=w405:string)  [unwired: 5 in, 1 out]
            n213 = call "Variables Data IO.vi"("Select"=Cmd_Var_Data_IO."Spec Old", "error in"=w408, "Data In"=w404, "Func_ext"=w405) -> ("error out"=w407:errorcluster)  [unwired: 5 in, 2 out]
            "Spec" <- w403
          }
        }
      }
      frame "측정방향변경" {
        w417 = 0 ("인덱스 (행)")
        n214 = property on="zero_30" class="Tbl (엄격한)"(error in=w414) -> (error out=w413:errorcluster, "Value"=w419:string[][], "DisabledEnum"=w420:T3)  [unwired: 1 in, 1 out]
        n215 = local read "Case"() -> (w422:enum16{"", "Case B", "Case D"})
        n216 = local read "zero_300"() -> (w424:string[][])
        n217 = Format Into String(w422) -> (resulting string=w423:string)  [unwired: 3 in, 1 out]
        n218 = case shown="\"Enabled\"" w420 {
          tunnel: w419 -> [_ w432]
          tunnel: ["ⅹ" w430] -> w418
          frame Default {
          }
          frame "Enabled" {
            w431 = 0 ("인덱스 (행)")
            n219 = Index Array(array=w432, index (row)=w431, index (col)=w431) -> (element=w430:string)
          }
        }
        n220 = Index Array(array=w424, index (row)=w417, index (col)=w417) -> (element=w416:string)
        n221 = Build Array(w418, w416, "측정방향", w423) -> (w415:string[])
        n222 = Build Array(w415) -> (w412:string[][])
        n223 = call "Variables Data IO.vi"("Select"=Cmd_Var_Data_IO."Result3", "error in"=w413, "Data In"=w412, "Func_ext"=w425) -> ("error out"=w426:errorcluster)  [unwired: 5 in, 2 out]
      }
    }
  }
  n224 = Release Queue(queue=w10, error in (no error)=w11) -> (error out=w8:errorcluster)  [unwired: 1 in, 2 out]
  n225 = Merge Errors(w9, w8) -> (→"에러 출력":errorcluster)
